vi "PostElogWithInlineImages.vi"() -> ()   [LabVIEW 2018]
uses:
  DataPacker/Utilities/ElogEncoding.ctl
  feGEM DataPacker.lvlib
panel:
  in  "Attributes (ie \nAuthor=Fred Dibna, \nSubject=Really important announcement)":string[](array[string])=["Subject=New feGEM elog tools!", "Author=Joseph", ""]
  out "Error Out":errorcluster
  in  "Elog Type (eg MicrowaveLog)":string="test"
  in  "Elog Encodeing":T1=enum."HTML"
  in  "HTML Message Part 2":string="<p>Above is a screenshot of the elog used to generate this post</p>\n<p>This example VI still requires the 'DataPacker' to be running somewhere in your project, and the maximum message size must be larger than the elog post you are making</p>\n<p>\n\n<p> This tool is not intended for causual usage, please dont spam attack the elog</p>"
  in  "Image to inline to elog post":path=path "ScreenshotOfThisTotallyWorkingFirstTime.png"
  in  "HTML Message Part 1":string="<h1>feGEM: Writing elogs from LabVIEW</h1>\n<p>The latest DataPacker is able to write elogs. This elog post was written and posted from labview.</p>\n<p>The intended use for this is for simple posts like the RWLog, or MicrowaveLog etc, however since this overhall you can post as plain text, clcode, or HTML. HTML involves more mark up but you can inline images directly into your post: "
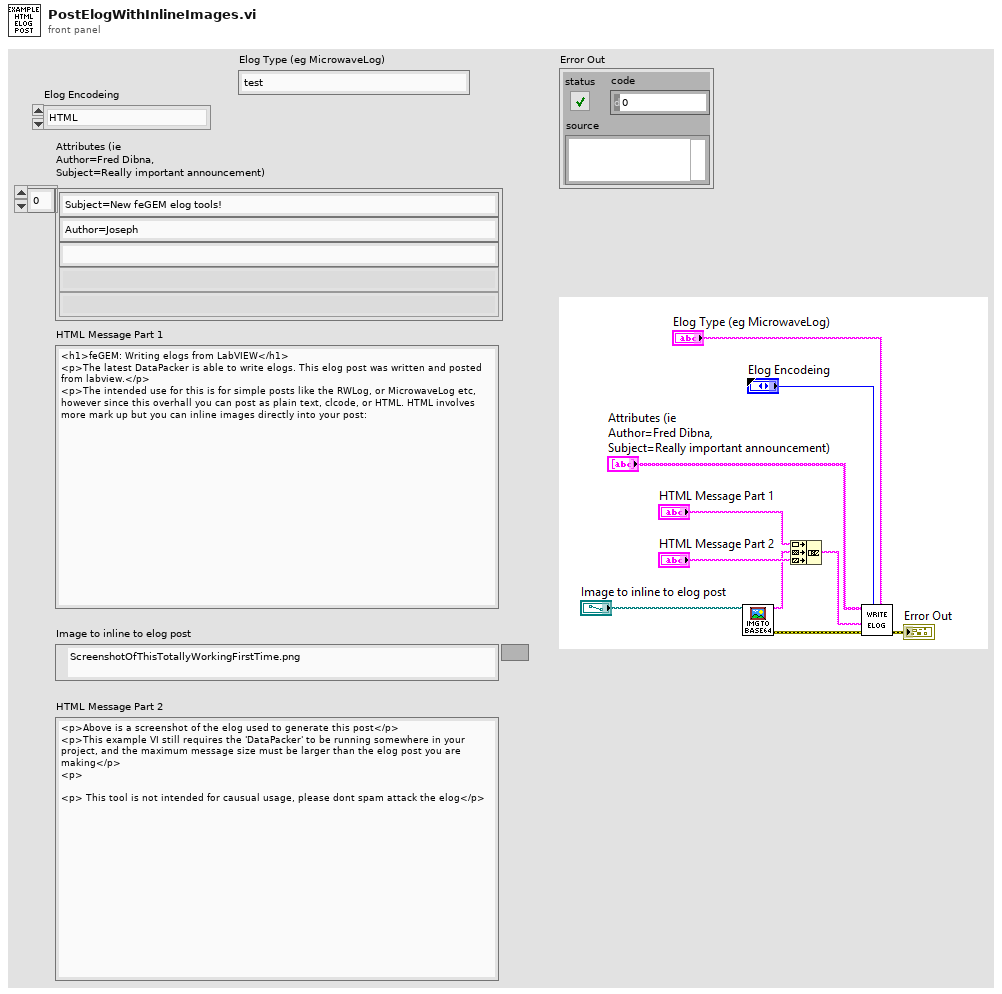
[diagram p1: front panel]
types:
  T1 = typedef "feGEM DataPacker.lvlib/ElogEncoding.ctl" = enum16{"ELCODE", "PLAIN", "HTML"}
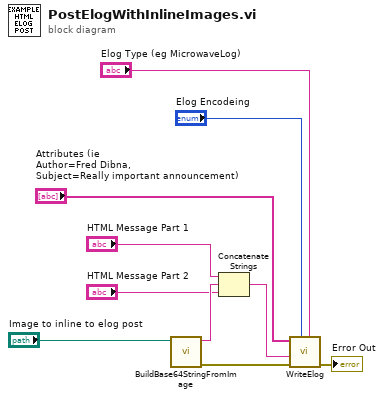
[diagram p0: block diagram]
diagram:
  n1 = call "BuildBase64StringFromImage.vi"("path"="Image to inline to elog post") -> ("error out"=w3:errorcluster, "concatenated string"=w8:string)  [unwired: 9 in]
  n2 = Concatenate Strings("HTML Message Part 1", w8, "HTML Message Part 2") -> (w4:string)
  n3 = call "WriteElog.vi"("Elog Type (eg MicrowaveLog)"="Elog Type (eg MicrowaveLog)", "Elog Encodeing"="Elog Encodeing", "error in (no error)"=w3, "Elog Message"=w4, "Attributes (ie \nAuthor=Fred Dibna, \nSubject=Really important announcement)"="Attributes (ie \nAuthor=Fred Dibna, \nSubject=Really important announcement)") -> ("Error Out"=→"Error Out":errorcluster)  [unwired: 6 in]
